vi "Script Rich to Flat Message Conversion.vi"(8 "error in (no error)":errorcluster, 9 "message metadata":T1, 10 "vi in":refnum<vi>, 11 "library in":refnum<vi>) -> (0 "error out":errorcluster, 2 "vi out":refnum<vi>, 3 "library out":refnum<vi>)   [LabVIEW 2019, in "gRPC Template Creation Utility.lvlib"]
uses:
  gRPC Template Creation Utility.lvlib
  TypeDefs/Message Metadata (Scripting).ctl
  TypeDefs/Message Element Metadata (Scripting).ctl
  TypeDefs/Message Element Type.ctl
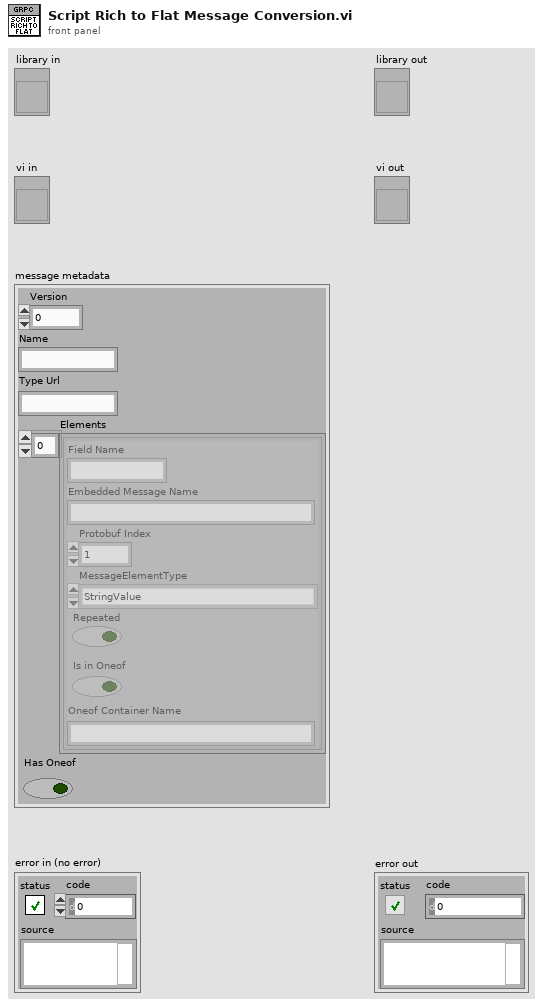
[diagram p1: front panel]
types:
  T1 = typedef "gRPC Template Creation Utility.lvlib/Message Metadata (Scripting).ctl" = cluster{"Version":i32, "Name":string, "Type Url":string, "Elements":T2[], "Has Oneof":bool}
  T2 = typedef "gRPC Template Creation Utility.lvlib/Message Element Metadata (Scripting).ctl" = cluster{"Field Name":string, "Embedded Message Name":string, "Protobuf Index":i32, "MessageElementType":T3, "Repeated":bool, "Is in Oneof":bool, "Oneof Container Name":string}
  T3 = typedef "gRPC Template Creation Utility.lvlib/Message Element Type.ctl" = enum32{"Int32Value", "FloatValue", "DoubleValue", "BoolValue", "StringValue", "MessageValue", "Int64Value", "UInt32Value", "UInt64Value", "EnumValue", "Bytes", "Fixed64", "Fixed32", "SFixed64", "SFixed32", "SInt64", "SInt32"}
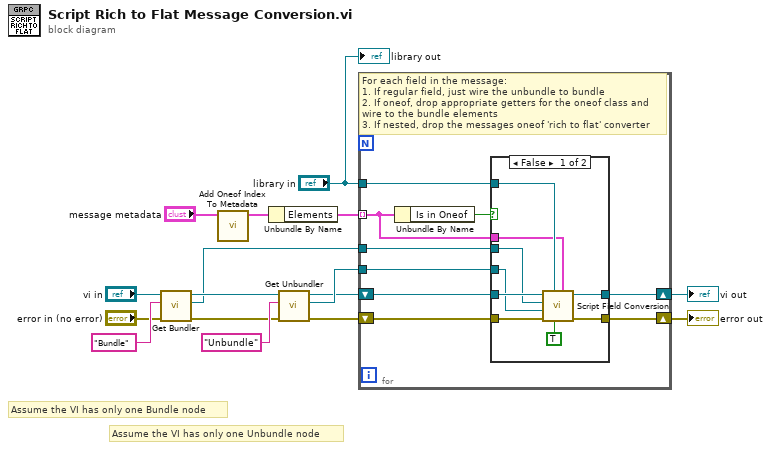
[diagram p0: block diagram]
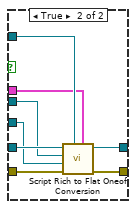
[diagram p2: hidden frame]
diagram:
  # "Assume the VI has only one Bundle node"
  # "Assume the VI has only one Unbundle node"
  n1 = call "Get Bundler.vi"("error in (no error)"="error in (no error)", "label"="Bundle" ("Class Name"), "owner vi in"="vi in") -> ("error out"=w7:errorcluster, "bundler ref"=w6:refnum<vi>, "owner vi out"=w8:refnum<vi>)  [unwired: 5 in, 1 out]
  n2 = call "Add Oneof Index To Metadata.vi"("message metadata"="message metadata") -> ("message metadata with oneof index"=w1:T1)  [unwired: 10 in]
  n3 = Unbundle By Name(w1) -> ("Elements"=w4:T2[])
  n4 = call "Get Unbundler.vi"("error in (no error)"=w7, "Label"="Unbundle" ("Class Name"), "Owner VI in"=w8) -> ("error out"=w5:errorcluster, "Unbundler Refnum"=w10:refnum<vi>, "Owner VI out"=w9:refnum<vi>)  [unwired: 5 in, 1 out]
  n5 = for {
    tunnel: w4 -> [w17] mode=indexing
    tunnel: w6 -> [w25]
    tunnel: w10 -> [w24]
    shift-right: [w21] -> w15
    shift-left: w5 -> [w20]
    shift-right: [w19] -> w16
    shift-left: w9 -> [w23]
    tunnel: "library in" -> [w22]
    # "For each field in the message:\n1. If regular field, just wire the unbundle to bundle\n2. If oneof, drop appropriate getters for the oneof class and wire to the bundle elements\n3. If nested, drop the messages oneof 'rich to flat' converter"
    n6 = Unbundle By Name(w17) -> ("Is in Oneof"=w18:bool)
    n7 = case shown="False" w18 {
      tunnel: w20 -> [w34 w42]
      tunnel: [w33 w41] -> w21
      tunnel: w25 -> [w29 w37]
      tunnel: w24 -> [w30 w38]
      tunnel: w23 -> [w32 w40]
      tunnel: w22 -> [w28 w36]
      tunnel: [w31 w39] -> w19
      tunnel: w17 -> [w27 w35]
      frame False {
        # "Wire unbundle and bundle nodes whose terminals have the same name across serialization and message cluster."
        n8 = call "Script Field Conversion.vi"("element metadata"=w27, "rich to flat"=TRUE, "library in"=w28, "error in (no error)"=w34, "unbundler"=w30, "bundler"=w29, "vi in"=w32) -> ("error out"=w33:errorcluster, "vi out"=w31:refnum<vi>)  [unwired: 3 in]
      }
      frame True {
        # "Get the bundle terminal whose name is <oneof container name>_selected_index.\nGet the unbundle terminal whose name is <oneof container name> which is the class terminal."
        n9 = call "Script Rich to Flat Oneof Conversion.vi"("element metadata"=w35, "library in"=w36, "error in (no error)"=w42, "unbundler"=w38, "bundler"=w37, "vi in"=w40) -> ("error out"=w41:errorcluster, "vi out"=w39:refnum<vi>)  [unwired: 4 in]
      }
    }
  }
  "error out" <- w15
  "vi out" <- w16
  "library out" <- "library in"
